vi "InitTrack.vi"(0 "AirSAS Controls in":T1 {"Waveform"."LFM Parameters"."Window %" format="%.2g"; "Waveform"."LFM Parameters"."Out. Amplitude (Vpk)" format="%0.2f"; "Waveform"."LFM Parameters"."Fstop (Hz)" format="%^.3e"; "Waveform"."LFM Parameters"."Fstart (Hz)" format="%^.3e"; "Waveform"."LFM Parameters"."Duration" format="%.3f"}, 2 "Vertical Min":dbl, 3 "error in (no error)":errorcluster) -> (6 "AirSAS Controls out":T1 {"Waveform"."LFM Parameters"."Window %" format="%.2g"; "Waveform"."LFM Parameters"."Out. Amplitude (Vpk)" format="%0.2f"; "Waveform"."LFM Parameters"."Fstop (Hz)" format="%^.3e"; "Waveform"."LFM Parameters"."Fstart (Hz)" format="%^.3e"; "Waveform"."LFM Parameters"."Duration" format="%.3f"}, 8 "output cluster":cluster{dbl, dbl, dbl}, 9 "error out":errorcluster)   [LabVIEW 2018]
uses:
  N:/SRDD-Student/Ng/fromTom/Air SAS Data Acquisition/controls/Air SAS Controls.ctl
  <vilib>/MakerHub/LINX/Private/Type Defs/LINX Ref.ctl
  <vilib>/MakerHub/LINX/Private/Type Defs/Platform.ctl
  <vilib>/MakerHub/LINX/Private/Type Defs/Interface.ctl
  <vilib>/MakerHub/LINX/Private/Device/Type Defs/LINX Device Config.ctl
  <vilib>/MakerHub/LINX/Private/Device/Type Defs/TCP Config.ctl
  <vilib>/MakerHub/LINX/Private/Device/Type Defs/Channels.ctl
  <vilib>/MakerHub/LINX/LMH-LINX.lvlib
  <vilib>/MakerHub/LINX/Private/Device/Device.lvlib
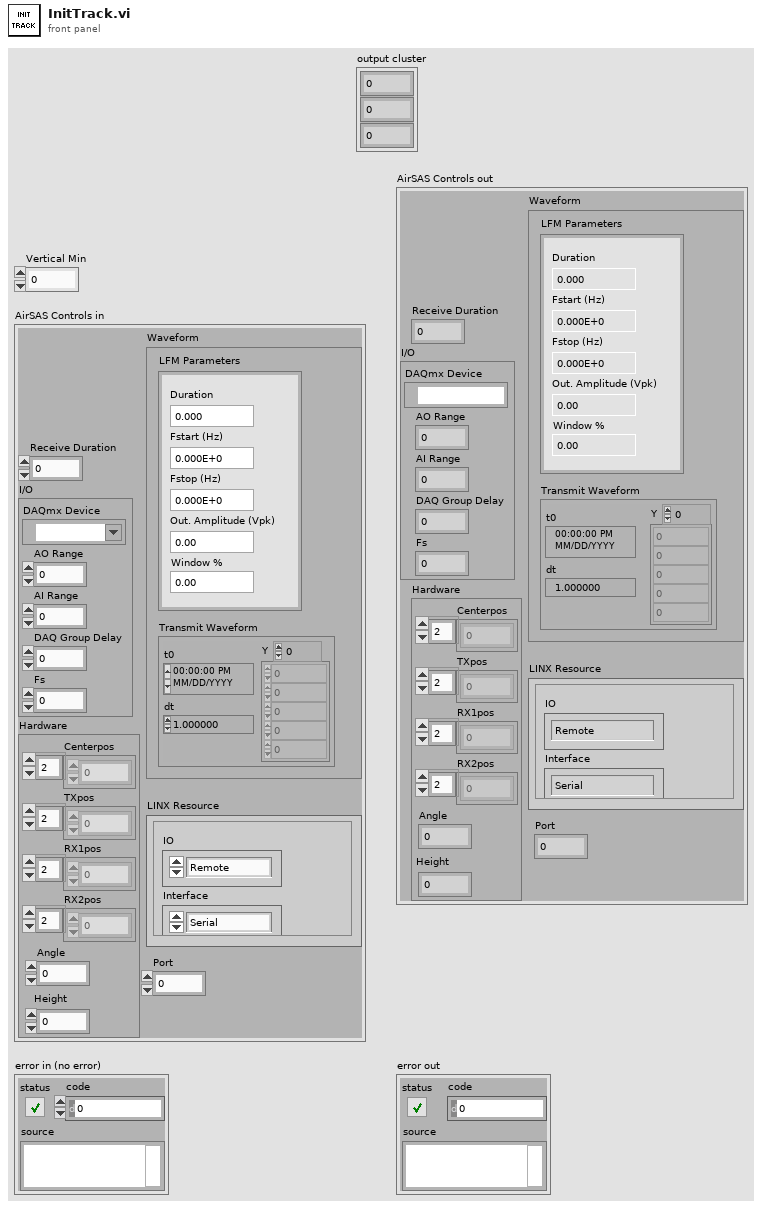
[diagram p1: front panel]
types:
  T1 = typedef "Air SAS Controls.ctl" = cluster{"Receive Duration":dbl, "I/O":cluster{"DAQmx Device":tag, "AO Range":dbl, "AI Range":dbl, "DAQ Group Delay":dbl, "Fs":dbl}, "Hardware":cluster{"Centerpos":dbl[], "TXpos":dbl[], "RX1pos":dbl[], "RX2pos":dbl[], "Angle":dbl, "Height":dbl}, "Waveform":cluster{"LFM Parameters":cluster{"Duration":dbl, "Fstart (Hz)":dbl, "Fstop (Hz)":dbl, "Out. Amplitude (Vpk)":dbl, "Window %":dbl}, "Transmit Waveform":waveform(dbl)}, "LINX Resource":T2, "Port":dbl}
  T2 = typedef "LMH-LINX.lvlib/LINX Ref.ctl" = cluster{"IO":T3, "Interface":T4, "LINX Device Config":T5}
  T3 = typedef "LMH-LINX.lvlib/Platform.ctl" = enum16{"Remote", "Local"}
  T4 = typedef "LMH-LINX.lvlib/Interface.ctl" = enum16{"Serial", "TCP"}
  T5 = typedef "LMH-LINX.lvlib/Device.lvlib/LINX Device Config.ctl" = cluster{"Interface":T4, "COM Port":refnum<visa-resource-name>, "TCP Configuration":T6, "Device Family":u8, "Device ID":u8, "Device Name":string, "TCP Ref":refnum<k5>, "Channels":T7}
  T6 = typedef "LMH-LINX.lvlib/Device.lvlib/TCP Config.ctl" = cluster{"IP Address":string, "Port":u16}
  T7 = typedef "LMH-LINX.lvlib/Channels.ctl" = cluster{"DI":u8[], "DO":u8[], "AI":u8[], "AO":u8[], "PWM":u8[], "QE":u8[], "UART":u8[], "I2C 2":u8[], "SPI":u8[], "CAN":u8[], "Servo":u8[], "AI Ref (V)":dbl, "AI Resolution (Bits)":u8, "AO Ref (V)":dbl, "AO Resolution (Bits)":u8}
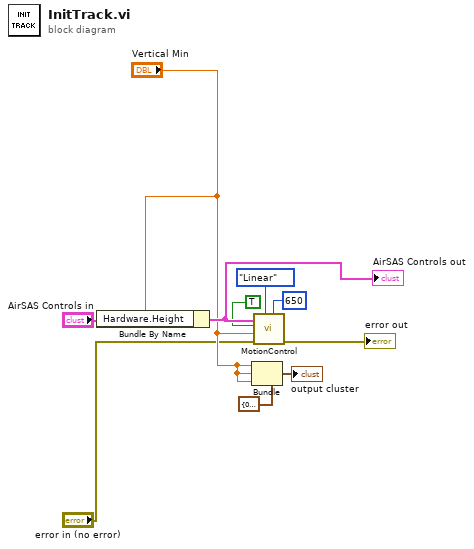
[diagram p0: block diagram]
diagram:
  n1 = Bundle By Name(cluster="AirSAS Controls in", "Hardware.Height"="Vertical Min") -> (w10:T1)
  "AirSAS Controls out" <- w10
  n2 = Bundle(cluster=cluster{dbl, dbl, dbl} {0.0, 227.2365805168986, 42.94234592445328} ("Slide 2"), "Vertical Min", "Vertical Min", "Vertical Min") -> (→"output cluster":cluster{dbl, dbl, dbl})
  n3 = call "MotionControl.vi"("Frequency (Hz) 3"=u32 650, "Motion Type"=enum16{"Linear", "Rotational"}."Linear", "Error In"="error in (no error)", "Distance"="Vertical Min", "Direction"=TRUE ("Boolean"), "AirSAS Controls"=w10) -> ("Error Out"=→"error out":errorcluster)  [unwired: 4 in, 1 out]
